vi "LSX Set Encoder Period.vi"(6 "dA":dbl, 7 "dZ":dbl, 8 "error in (no error)":errorcluster, 9 "dY":dbl, 10 "dX":dbl, 11 "lLSID":i32) -> (0 "error out":errorcluster, 3 "function return":i32)   [LabVIEW 2018, in "Tango.lvlib"]
doc: "TANGOAPI int TANGOCALL LSX_SetEncoderPeriod (int lLSID, double dX, double dY, double dZ, double dA);"
uses:
  <userlib>/Tango/Tango.lvlib
  <userlib>/Tango/Tango_DLL.dll
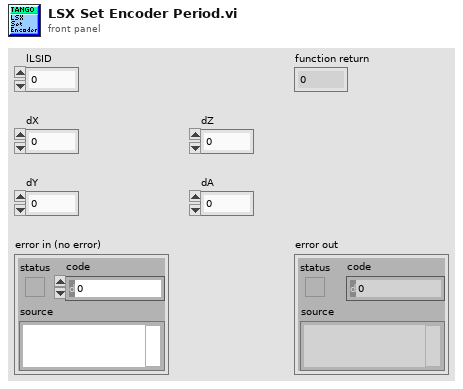
[diagram p1: front panel]
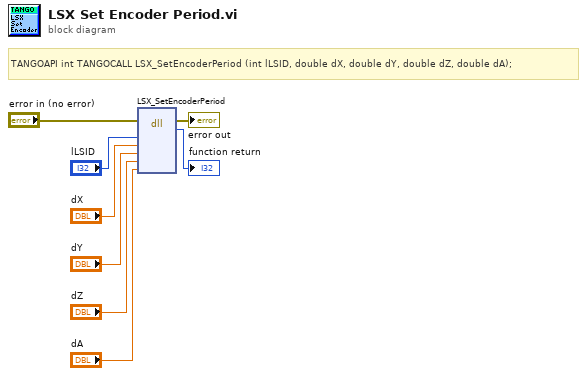
[diagram p0: block diagram]
diagram:
  # "TANGOAPI int TANGOCALL LSX_SetEncoderPeriod (int lLSID, double dX, double dY, double dZ, double dA);"
  n1 = dll-call lib="C:/Program Files (x86)/National Instruments/LabVIEW 2018/user.lib/Tango/Tango_DLL.*" fn="LSX_SetEncoderPeriod"(error in="error in (no error)", "lLSID"="lLSID", "dX"="dX", "dY"="dY", "dZ"="dZ", "dA"="dA") -> (error out=→"error out":errorcluster, →"function return":i32)  [unwired: 7 in, 1 out]
